vi "AB_Set_Destination_Type.vi"(8 "error in (no error)":errorcluster, 9 "destination type":T1, 10 "destination index":i32, 11 "destinations in":refnum<class "AB_Destination.lvclass">[](array[class])) -> (0 "error out":errorcluster, 2 "Destination path":path, 3 "destinations out":refnum<class "AB_Destination.lvclass">[](array[class]))   [LabVIEW 2020]
uses:
  <vilib>/AppBuilder/AB_Classes/Destination/AB_Destination.lvclass
  <vilib>/AppBuilder/AB_Destination_Type.ctl
  <vilib>/AppBuilder/AB_Classes/Destination/Dest_LLB/AB_Dest_LLB.lvclass
  e:/builds/penguin/labview/branches/2020/dev/dist/vi.lib/AppBuilder/AB_Classes/Destination/AB_Destination.lvclass
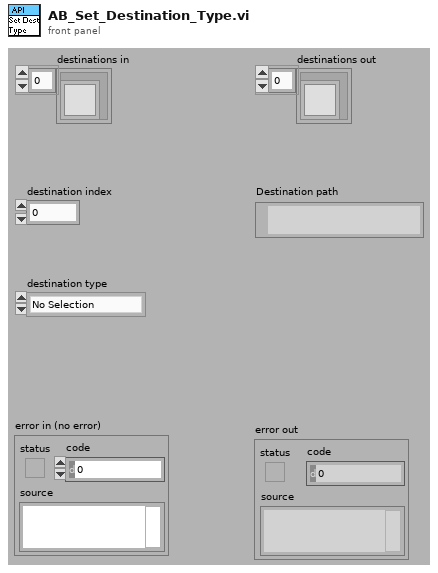
[diagram p1: front panel]
types:
  T1 = typedef "AB_Destination_Type.ctl" = enum32{"No Selection", "Directory", "LLB"}
  T2 = typedef "AB_Destination.ctl" = cluster{"destName":string, "path":path, "libraryName":string, "preserveHierarchy":bool, "eng_inBuild":bool, "eng_libraryReference":refnum<vi>, "eng_restictAddToNewLibrary":bool}
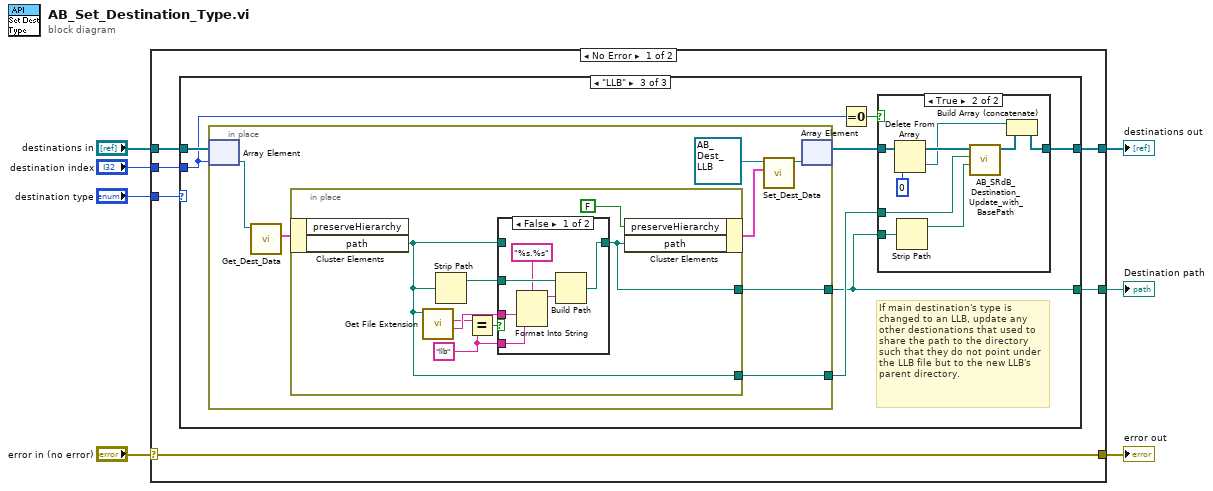
[diagram p0: block diagram]
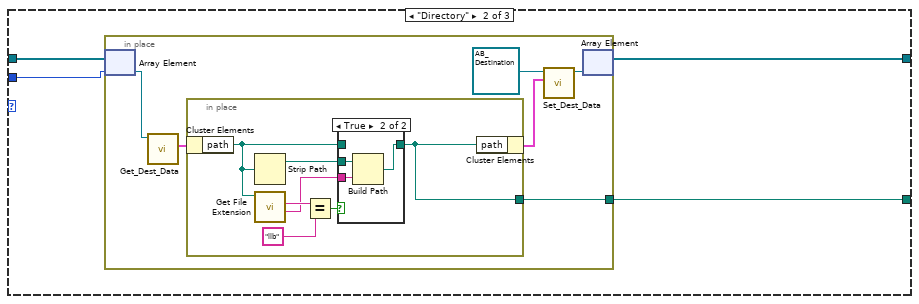
[diagram p3: hidden frame]
diagram:
  n1 = case shown="No Error" "error in (no error)" {
    selector: "error in (no error)" -> [w9 w76]
    tunnel: [w9 w76] -> w6
    tunnel: "destinations in" -> [w13 w75]
    tunnel: "destination index" -> [w12 _]
    tunnel: [w11 w75] -> w3
    tunnel: [w10 _] -> w2
    tunnel: "destination type" -> [w8 _]
    frame No Error {
      n2 = case shown="\"LLB\"" w8 {
        tunnel: w13 -> [w14 w18 w42]
        tunnel: w12 -> [_ w15 w41]
        tunnel: [w14 w17 w38] -> w11
        tunnel: [_ w16 w36] -> w10
        frame "No Selection" {
        }
        frame "Directory" {
          n3 = in-place {
            in-place-border: [w19] -> w16
            n4 = in-place-array #1(w18, w15) -> (w20:refnum<class "AB_Destination.lvclass">)
            n5 = call <vilib>:"Get_Dest_Data.vi"("Class in"=w20) -> ("destName"=w23:T2)  [unwired: 1 in, 9 out]
            n6 = in-place {
              in-place-border: [w25] -> w19
              n7 = in-place-cluster #2(w23) -> ("path"=w26:path)
              n8 = Strip Path(path=w26) -> (stripped path=w31:path)  [unwired: 1 out]
              n9 = call <vilib>:"Get File Extension.vi"("file"=w26) -> ("filename without extension"=w27:string, "lowercase file extension"=w28:string)  [unwired: 1 in, 8 out]
              n10 = Equal?(x=w28, y="llb") -> (x = y?=w29:bool)
              n11 = case shown="True" w29 {
                tunnel: w31 -> [_ w35]
                tunnel: w27 -> [_ w34]
                tunnel: [w32 w33] -> w25
                tunnel: w26 -> [w32 _]
                frame False {
                }
                frame True {
                  n12 = Build Path(base path=w35, name or relative path=w34) -> (appended path=w33:path)
                }
              }
              n13 = in-place-cluster #2("path"=w25) -> (w22:T2)
            }
            n14 = call <vilib>:"Set_Dest_Data.vi"("destName"=w22, "Class in"=refnum<class "AB_Destination.lvclass"> refnum ("AB_Destination.lvclass")) -> ("Class out"=w21:refnum<class "AB_Destination.lvclass">)  [unwired: 1 in, 8 out]
            n15 = in-place-array #1(w21) -> (w17:refnum<class "AB_Destination.lvclass">[])  [unwired: 1 out]
          }
        }
        frame "LLB" {
          # "If main destination's type is changed to an LLB, update any other destionations that used to share the path to the directory such that they do not point under the LLB file but to the new LLB's parent directory."
          n16 = in-place {
            in-place-border: [w54] -> w36
            in-place-border: [w53] -> w37
            n17 = in-place-array #3(w42, w41) -> (w56:refnum<class "AB_Destination.lvclass">)
            n18 = call <vilib>:"Get_Dest_Data.vi"("Class in"=w56) -> ("destName"=w59:T2)  [unwired: 1 in, 9 out]
            n19 = in-place {
              in-place-border: [w61] -> w54
              in-place-border: [w60] -> w53
              w65 = "llb" ("y")
              n20 = in-place-cluster #4(w59) -> ("path"=w60:path)  [unwired: 1 out]
              n21 = call <vilib>:"Get File Extension.vi"("file"=w60) -> ("filename without extension"=w67:string, "lowercase file extension"=w66:string)  [unwired: 1 in, 8 out]
              n22 = Strip Path(path=w60) -> (stripped path=w63:path)  [unwired: 1 out]
              n23 = Equal?(x=w66, y=w65) -> (x = y?=w64:bool)
              n24 = case shown="False" w64 {
                tunnel: w63 -> [w73 _]
                tunnel: [w72 w74] -> w61
                tunnel: w60 -> [_ w74]
                tunnel: w67 -> [w70 _]
                tunnel: w65 -> [w69 _]
                frame False {
                  n25 = Format Into String(format string="%s.%s", w70, w69) -> (resulting string=w68:string)  [unwired: 2 in, 1 out]
                  n26 = Build Path(base path=w73, name or relative path=w68) -> (appended path=w72:path)
                }
                frame True {
                }
              }
              n27 = in-place-cluster #4("preserveHierarchy"=FALSE, "path"=w61) -> (w58:T2)
            }
            n28 = call <vilib>:"Set_Dest_Data.vi"("destName"=w58, "Class in"=refnum<class "AB_Dest_LLB.lvclass"> refnum ("AB_Dest_LLB.lvclass")) -> ("Class out"=w57:refnum<class "AB_Dest_LLB.lvclass">)  [unwired: 1 in, 8 out]
            n29 = in-place-array #3(w57) -> (w40:refnum<class "AB_Destination.lvclass">[])  [unwired: 1 out]
          }
          n30 = Equal To 0?(x=w41) -> (x = 0?=w39:bool)
          n31 = case shown="True" w39 {
            tunnel: w40 -> [w43 w49]
            tunnel: [w43 w44] -> w38
            tunnel: w37 -> [_ w52]
            tunnel: w36 -> [_ w51]
            frame False {
            }
            frame True {
              n32 = Delete From Array(array=w49, index=0) -> (deleted portion=w46:refnum<class "AB_Destination.lvclass">, array with subset deleted=w48:refnum<class "AB_Destination.lvclass">[])  [unwired: 1 in]
              n33 = Strip Path(path=w51) -> (stripped path=w50:path)  [unwired: 1 out]
              n34 = call <resource>:"AB_SRdB_Destination_Update_with_BasePath.vi"("new base path"=w50, "old base path"=w52, "ALL data in"=w48) -> ("ALL data out"=w45:refnum<class "AB_Destination.lvclass">[])  [unwired: 7 in, 1 out]
              n35 = Build Array (concatenate)(w46, w45) -> (w44:refnum<class "AB_Destination.lvclass">[])
            }
          }
        }
      }
    }
    frame Error {
    }
  }
  "error out" <- w6
  "Destination path" <- w2
  "destinations out" <- w3
